vi "PathPlanner_PathFinder_Globals.vi"() -> ()   [LabVIEW 2019, in "PathPlanner24.lvlib"]
doc: "Globals for Path FInder"
uses:
  PathPlanner24.lvlib
  TypeDef/PathPlannerObstacleGrid.ctl
  <vilib>/Rock Robotics/WPI/ThirdParty/JAS_Junk/TrajLib/TypeDef/TRANSLATION2D.ctl
  TypeDef/PathPlannerFinderGridPosition.ctl
  <vilib>/robotics/Navigation/shared/WorldMap/OccupancyGridWorldMap/NI_Robotics_OccupancyGridWorldMap.lvclass
  TypeDef/PathPlannerFinderDoublePair.ctl
  <vilib>/robotics/Navigation/Anytime D Star/NI_Robotics_AnytimeDStar.lvclass
  <vilib>/robotics/Navigation/shared/MapNode/OccupancyGridNode/NI_Robotics_OccupancyGridMapNode.lvclass
  <vilib>/robotics/Navigation/shared/MapNode/AbstractDstarNode/NI_Robotics_AbstractDstarNode.lvclass
  <vilib>/Rock Robotics/WPI/ThirdParty/JAS_Junk/TrajLib/Trajectory_Library.lvlib
panel:
  out "ExtractedFieldPosPath":T1[](array[typedef]) {"Y" step=0.25 format="%14.3f"; "X" format="%14.3f"}
  out "path references":refnum<data-value>[](array[refnum])
  out "DoMajorErrCount":i64
  out "DoMinorErrCount":i64
  out "DoResetErrCount":i64
  out "Goal Cell Ref":refnum<data-value>
  out "Start Cell Ref":refnum<data-value>
  out "PathFind ADStar":refnum<class "NI_Robotics_AnytimeDStar.lvclass">
  out "ExtractedPathSimplified":T2[](array[typedef])
  out "ExtractedPath":T2[](array[typedef])
  out "DoMajorCount":i64
  out "DoMinorCount":i64
  out "DoResetCount":i64
  out "DoWorkLoopCount":i64
  out "Main Program Name":string
  out "WorkQueue":refnum<queue>
  out "Incons":map{i32, T3}(c390)
  out "Open":map{i32, T3}(c390)
  out "Rhs":map{i32, dbl}(c390)
  out "G":map{i32, dbl}(c390)
  out "eps_little":dbl
  out "Closed":set{T2}(c389)
  out "DynamicObstacles":set{T2}(c389)
  out "Obstacles":set{T2}(c389)
  out "StaticObstacles":set{T2}(c389)
  out "StaticOccupancyGrid":refnum<data-value>
  in  "SGoal":T2
  in  "SStart":T2
  out "NodeSize_M":dbl=0.2
  out "FieldWidth_M":dbl=8.02
  out "FieldLength_M":dbl=16.54
  out "NodesY":i32
  out "NodesX":i32
  in  "CurrentPath":T1[](array[typedef]) {"Y" format="%14.3f"; "X" format="%14.3f"}
  out "TerminateWorker":bool
  out "NewPathAvailLastCheck":i32
  out "NewPathAvailCount":i32
  in  "RealGoalPosition":T1 {"Y" format="%14.3f"; "X" format="%14.3f"}
  in  "RealStartPosition":T1 {"Y" format="%14.3f"; "X" format="%14.3f"}
  out "PathPlanner_ObstacleGrid":T4
  out "BackGroundInitialized":bool
  # "debug"
  # "Worker initializes these"
  # "Only for port of PathPlanner AD Star"
  # "For LabVIEW AD Star"
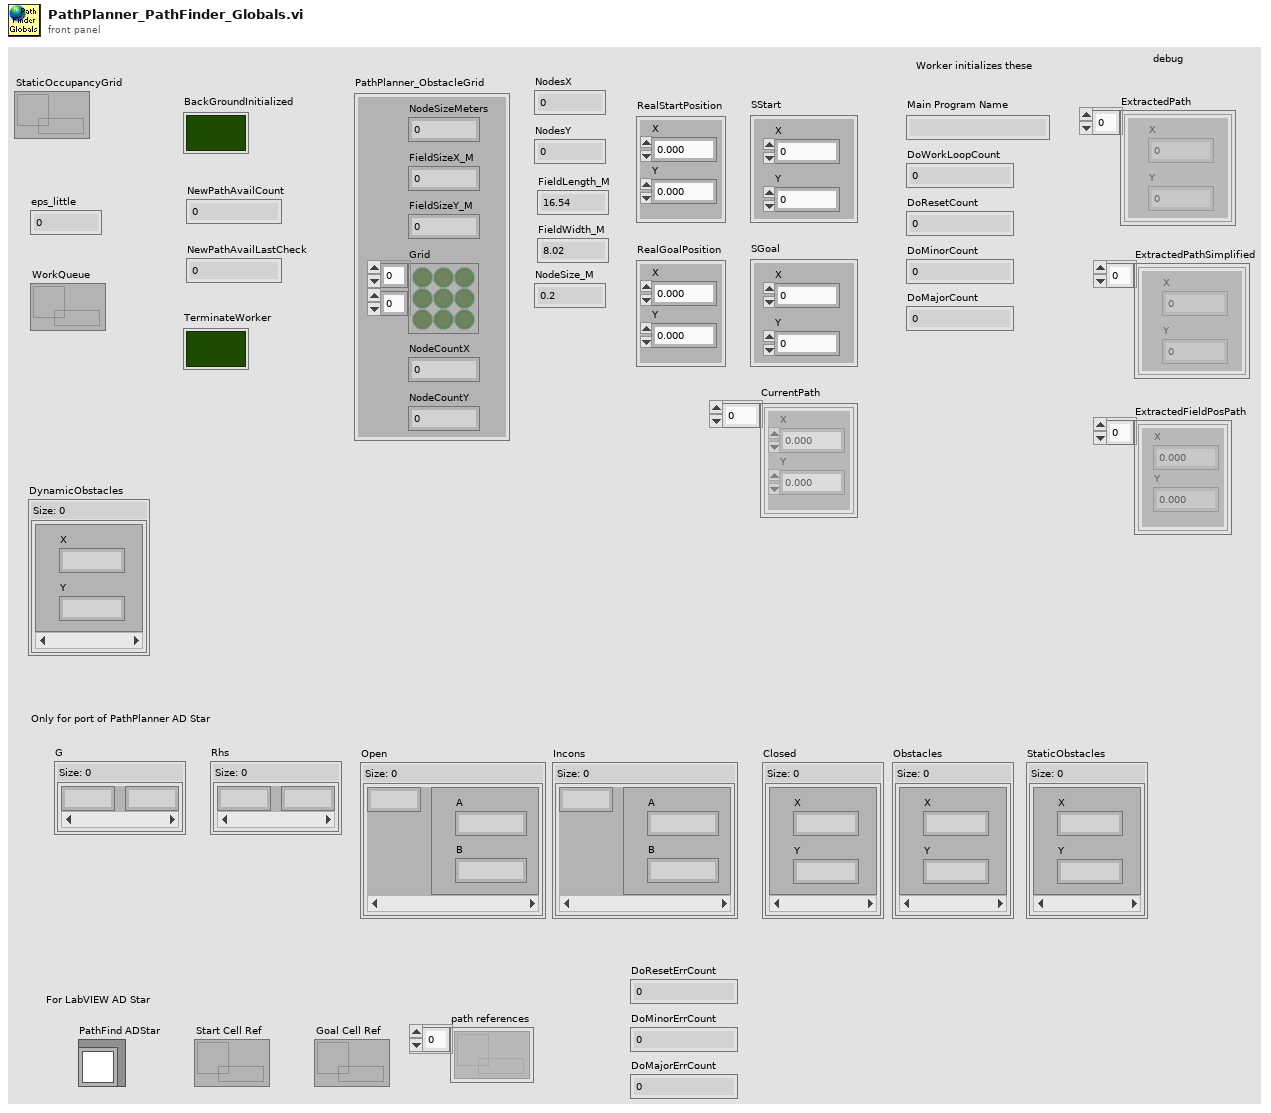
[diagram p1: front panel]
types:
  T1 = typedef "Trajectory_Library.lvlib/TRANSLATION2D.ctl" = cluster{"X":dbl, "Y":dbl}
  T2 = typedef "PathPlanner24.lvlib/PathPlannerFinderGridPosition.ctl" = cluster{"X":i32, "Y":i32}
  T3 = typedef "PathPlanner24.lvlib/PathPlannerFinderDoublePair.ctl" = cluster{"A":dbl, "B":dbl}
  T4 = typedef "PathPlanner24.lvlib/PathPlannerObstacleGrid.ctl" = cluster{"NodeSizeMeters":dbl, "Grid":bool[][], "NodeCountX":i32, "NodeCountY":i32, "FieldSizeX_M":dbl, "FieldSizeY_M":dbl}
diagram:
